vi "refgen.vi"(7 "refgen":cluster{"slope":dbl, "period":dbl}, 11 "Qube":refnum<class "Qube.lvclass">) -> (1 "r":dbl, 3 "Qube":refnum<class "Qube.lvclass">)   [LabVIEW 2020, in "Qube.lvclass"]
uses:
  Qube.lvclass
  Qube.lvclass/Qube.ctl
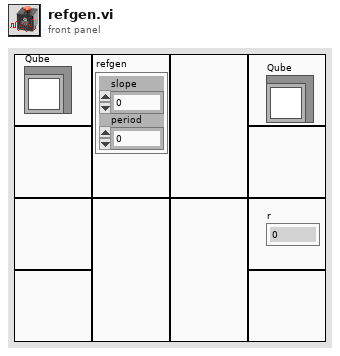
[diagram p1: front panel]
types:
  T1 = typedef "Qube.lvclass/mode.ctl" = enum16{"Control", "Identify"}
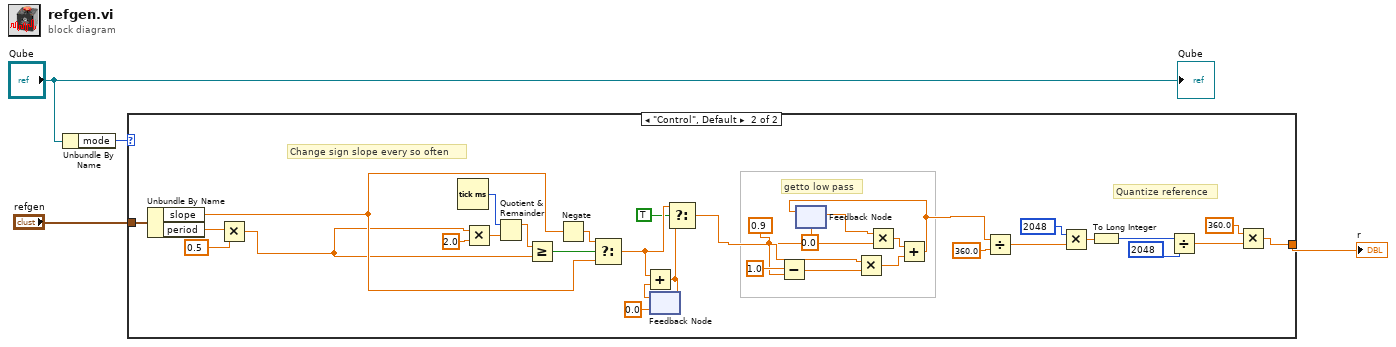
[diagram p0: block diagram]
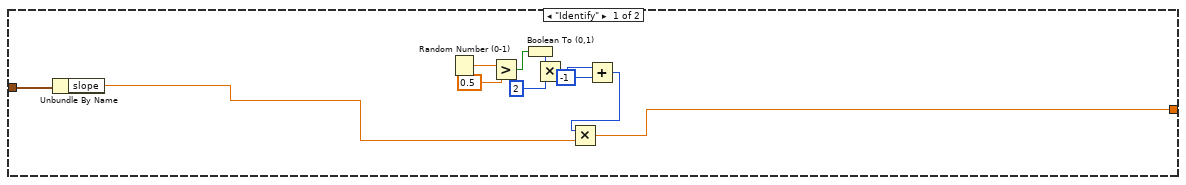
[diagram p2: hidden frame]
diagram:
  n1 = Unbundle By Name("Qube") -> ("mode"=w3:T1)
  n2 = case shown="\"Control\", Default" w3 {
    tunnel: [w5 w20] -> w4
    tunnel: "refgen" -> [w15 w49]
    frame "Identify" {
      n3 = Unbundle By Name(w15) -> ("slope"=w6:dbl)
      n4 = Random Number (0-1)() -> (number: 0 to 1=w14:dbl)
      n5 = Greater?(x=w14, y=0.5) -> (0:w12:bool)
      n6 = Boolean To (0,1)(Boolean=w12) -> (0, 1=w11:i16)
      n7 = Multiply(x=w11, y=i16 2) -> (x*y=w10:i16)
      n8 = Add(x=w10, y=i16 -1) -> (x+y=w7:i16)
      n9 = Multiply(x=w7, y=w6) -> (x*y=w5:dbl)
    }
    frame "Control", Default {
      w17 = 0.9 ("y")
      # "Quantize reference"
      # "getto low pass"
      # "Change sign slope every so often"
      n10 = Unbundle By Name(w49) -> ("slope"=w42:dbl, "period"=w41:dbl)
      n11 = Multiply(x=w41, y=0.5) -> (x*y=w37:dbl)
      n12 = Tick Count (ms)() -> (millisecond timer value=w48:u32)
      n13 = Multiply(x=w37, y=2.0) -> (x*y=w47:dbl)
      n14 = Quotient & Remainder(x=w48, y=w47) -> (x-y*floor(x/y)=w45:dbl)  [unwired: 1 out]
      n15 = Greater Or Equal?(x=w45, y=w37) -> (x >= y?=w44:bool)
      n16 = Negate(x=w42) -> (-x=w43:dbl)
      n17 = Select(t=w43, s=w44, f=w42) -> (s? t:f=w35:dbl)
      n18 = feedback #1(0.0) -> (w39:dbl)
      n19 = Add(x=w35, y=w39) -> (x+y=w36:dbl)
      n20 = feedback-in #1(w36) -> ()
      n21 = Select(t=w35, s=TRUE, f=w36) -> (s? t:f=w29:dbl)
      n22 = Subtract(x=1.0, y=w17) -> (x-y=w16:dbl)
      n23 = feedback #2(0.0) -> (w33:dbl)
      n24 = Multiply(x=w29, y=w16) -> (x*y=w31:dbl)
      n25 = Multiply(x=w33, y=w17) -> (x*y=w32:dbl)
      n26 = Add(x=w32, y=w31) -> (x+y=w19:dbl)
      n27 = feedback-in #2(w19) -> ()
      n28 = Divide(x=w19, y=360.0) -> (x/y=w26:dbl)
      n29 = Multiply(x=2048 ("y"), y=w26) -> (x*y=w27:dbl)
      n30 = To Long Integer(number=w27) -> (32bit integer=w28:i32)
      n31 = Divide(x=w28, y=2048) -> (x/y=w25:dbl)
      n32 = Multiply(x=360.0, y=w25) -> (x*y=w20:dbl)
    }
  }
  "r" <- w4
  "Qube" <- "Qube"
